vi "Triangle Demo Init.vi"() -> (3 "Array":refnum<class "Shape.lvclass">[](array[class]))   [LabVIEW 2015]
uses:
  Shape/Shape.lvclass
  Circle/Circle.lvclass
  Square/Square.lvclass
  colors.ctl
  Circle/Circle.lvclass/Circle.ctl
  Shape/Shape.lvclass/Shape.ctl
  Square/Square.lvclass/Square.ctl
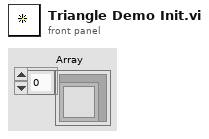
[diagram p1: front panel]
types:
  T1 = typedef "colors.ctl" = enum16{"Blue", "Red", "Green", "Yellow"}
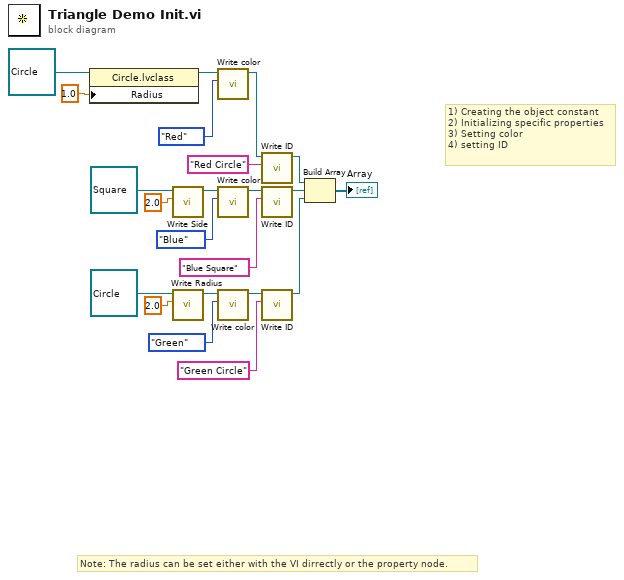
[diagram p0: block diagram]
diagram:
  # "1) Creating the object constant\n2) Initializing specific properties\n3) Setting color\n4) setting ID"
  # "Note: The radius can be set either with the VI dirrectly or the property node."
  n1 = property class="Circle.lvclass"(reference=refnum<class "Circle.lvclass"> refnum ("Circle.lvclass"), "Radius"=1.0) -> (reference out=w20:refnum<class "Circle.lvclass">)  [unwired: 1 in, 1 out]
  n2 = call "Write Side.vi"("Side"=2.0, "Square in"=refnum<class "Square.lvclass"> refnum ("Square.lvclass")) -> ("Square out"=w12:refnum<class "Square.lvclass">)  [unwired: 8 in, 1 out]
  n3 = call "Write Radius.vi"("Radius"=2.0, "Circle in"=refnum<class "Circle.lvclass"> refnum ("Circle.lvclass")) -> ("Circle out"=w2:refnum<class "Circle.lvclass">)  [unwired: 8 in, 1 out]
  n4 = call "Write color.vi"("color"=colors."Red", "Shape in"=w20) -> ("Shape out"=w22:refnum<class "Circle.lvclass">)  [unwired: 8 in, 1 out]
  n5 = call "Write color.vi"("color"=colors."Blue", "Shape in"=w12) -> ("Shape out"=w13:refnum<class "Square.lvclass">)  [unwired: 8 in, 1 out]
  n6 = call "Write color.vi"("color"=colors."Green", "Shape in"=w2) -> ("Shape out"=w17:refnum<class "Circle.lvclass">)  [unwired: 8 in, 1 out]
  n7 = call "Write ID.vi"("ID"="Red Circle", "Shape in"=w22) -> ("Shape out"=w18:refnum<class "Circle.lvclass">)  [unwired: 8 in, 1 out]
  n8 = call "Write ID.vi"("ID"="Blue Square", "Shape in"=w13) -> ("Shape out"=w15:refnum<class "Square.lvclass">)  [unwired: 8 in, 1 out]
  n9 = call "Write ID.vi"("ID"="Green Circle", "Shape in"=w17) -> ("Shape out"=w14:refnum<class "Circle.lvclass">)  [unwired: 8 in, 1 out]
  n10 = Build Array(w18, w15, w14) -> (→"Array":refnum<class "Shape.lvclass">[])
